vi "单通道测试.vi"() -> ()   [LabVIEW 2015]
panel:
  in  "Limit":dbl=1.0
  out "消息":string
  in  "stop":bool
  in  "测试类型":enum32{"直通基准", "校准基准", "校准测试"}(radio)
  in  "测试":bool
  in  "out":i32=1
  in  "in":i32=1
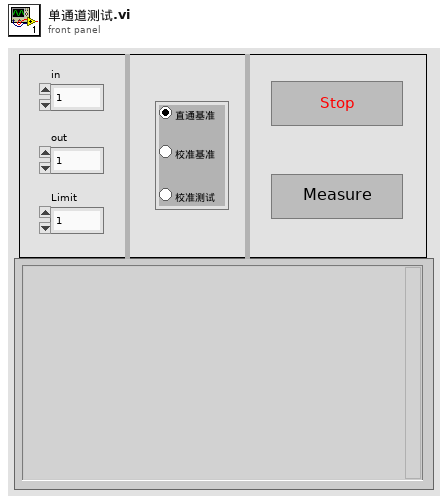
[diagram p1: front panel]
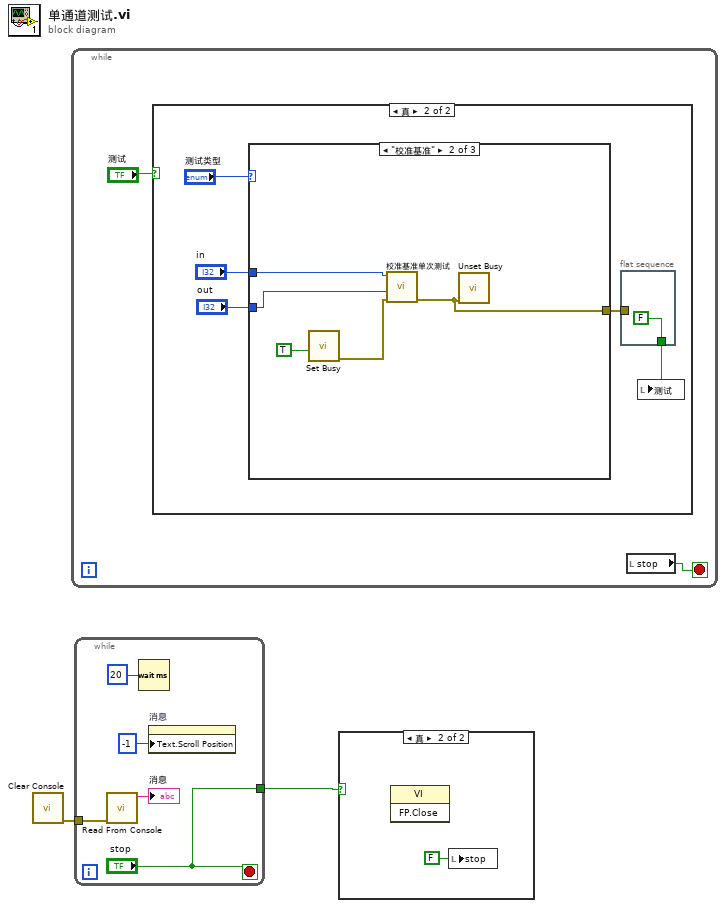
[diagram p0: block diagram]
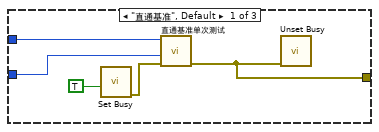
[diagram p4: hidden frame]
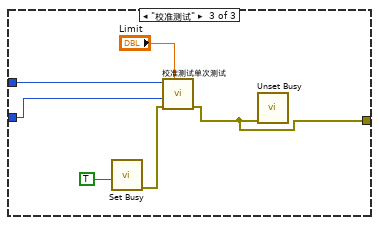
[diagram p5: hidden frame]
diagram:
  n1 = call "Clear Console.vi"() -> ("error out"=w1:errorcluster)  [unwired: 11 in]
  n2 = while {
    stop <- w3 stop-if-true
    n3 = case shown="真" "测试" {
      frame False {
      }
      frame True {
        n4 = case shown="\"校准基准\"" "测试类型" {
          tunnel: "in" -> [w15 w19 w25]
          tunnel: "out" -> [w14 w18 w24]
          tunnel: [w11 w16 w21] -> w6
          frame "直通基准", Default {
            n5 = call <vilib>:"Set Busy.vi"("disable click? (T)"=TRUE) -> ("error out"=w12:errorcluster)  [unwired: 9 in, 1 out]
            n6 = call "直通基准单次测试.vi"("error in"=w12, "out"=w14, "in"=w15) -> ("error out"=w11:errorcluster)  [unwired: 8 in]
            n7 = call <vilib>:"Unset Busy.vi"("error in (no error)"=w11) -> ()  [unwired: 10 in, 1 out]
          }
          frame "校准基准" {
            n8 = call <vilib>:"Set Busy.vi"("disable click? (T)"=TRUE) -> ("error out"=w17:errorcluster)  [unwired: 9 in, 1 out]
            n9 = call "校准基准单次测试.vi"("error in"=w17, "out"=w18, "in"=w19) -> ("error out"=w16:errorcluster)  [unwired: 8 in]
            n10 = call <vilib>:"Unset Busy.vi"("error in (no error)"=w16) -> ()  [unwired: 10 in, 1 out]
          }
          frame "校准测试" {
            n11 = call <vilib>:"Set Busy.vi"("disable click? (T)"=TRUE) -> ("error out"=w23:errorcluster)  [unwired: 9 in, 1 out]
            n12 = call "校准测试单次测试.vi"("Limit"="Limit", "error in (no error)"=w23, "out"=w24, "in"=w25) -> ("error out"=w21:errorcluster)  [unwired: 7 in]
            n13 = call <vilib>:"Unset Busy.vi"("error in (no error)"=w21) -> ()  [unwired: 10 in, 1 out]
          }
        }
        n14 = flat-sequence {
          tunnel: w6 -> [_]
          tunnel: [FALSE] -> w5
          frame #0 {
          }
        }
        n15 = local write "测试"(w5) -> ()
      }
    }
    n16 = local read "stop"() -> (w3:bool)
  }
  n17 = while {
    tunnel: w1 -> [w30]
    tunnel: ["stop"] -> w2
    stop <- "stop" stop-if-true
    n18 = call "Read From Console.vi"("error in (no error)"=w30) -> ("Output"=→"消息":string)  [unwired: 9 in, 1 out]
    n19 = Wait (ms)(milliseconds to wait=u32 20) -> ()  [unwired: 1 out]
    n20 = property on="消息" class="Str"("Text.Scroll Position"=i8 -1 ("milliseconds to wait")) -> ()  [unwired: 2 in, 2 out]
  }
  n21 = case shown="真" w2 {
    frame False {
    }
    frame True {
      n22 = invoke class="VI" method="FP.Close"() -> ()  [unwired: 3 in, 3 out]
      n23 = local write "stop"(FALSE ("stop")) -> ()
    }
  }
